vi "Process.vi"() -> ()   [LabVIEW 2020, in "RTAF.lvlib" / "System Status Actor.lvclass"]
uses:
  System Status Actor.lvclass
  Status.ctl
  Total Used Free MB.ctl
  Base Actor/Actor/Actor.lvclass/Actor.ctl
  Base Actor/Sequencer/Sequencer.lvclass/Sequencer.ctl
  System Status Actor.lvclass/System Status Actor.ctl
  C:/dev/PGS/2001 - TBCM/Source/RT/RTAF/Source/RTAF/Actors/Base Actor/Actor/Actor.lvclass
  API/System Status Actor API.lvclass
  <vilib>/Utility/High Resolution Relative Seconds.vi
  Global References.vi
  Base Actor/Actor/Actor.lvclass
  C:/dev/PGS/2001 - TBCM/Source/RT/RTAF/Source/RTAF/Actors/System Status/Actor/System Status Actor.lvclass
  RTAF.lvlib
panel:
  out "Status":T1 {"Uptime" format="%<%H:%M:%S%1u>t"}
  out "Iteration":i32
  in  "Tick Period [ms]":i32=5 min=2 step=1
  out "Tick Period [s]":dbl format="%.1p"
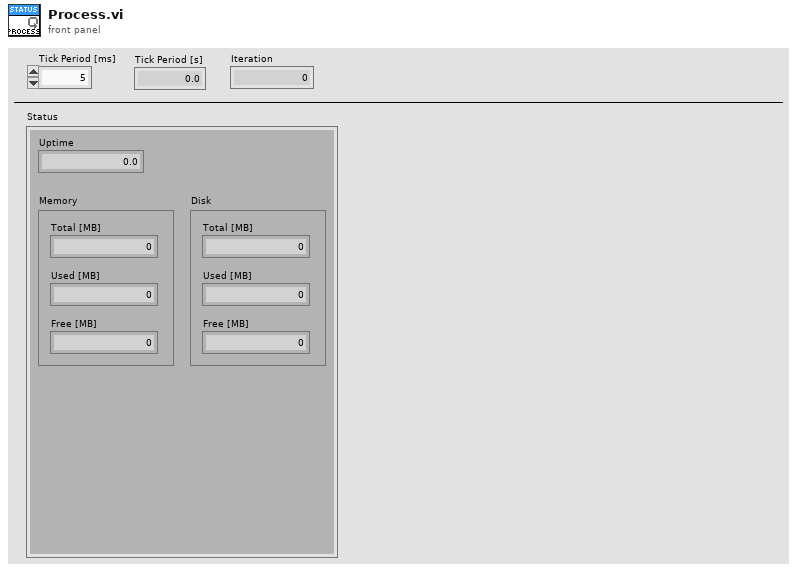
[diagram p1: front panel]
types:
  T1 = typedef "RTAF.lvlib/System Status Actor.lvclass/Status.ctl" = cluster{"Memory":T2, "Disk":T2, "Uptime":dbl}
  T2 = typedef "RTAF.lvlib/System Status Actor.lvclass/Total Used Free MB.ctl" = cluster{"Total [MB]":dbl, "Used [MB]":dbl, "Free [MB]":dbl}
  T3 = typedef "RTAF.lvlib/System Status Actor.lvclass/Mailboxes.ctl" = cluster{"Instructions":refnum<event-registration>}
  T4 = enum32{"Invalid", "Standard", "Closed", "Hidden", "Minimized", "Maximized"}
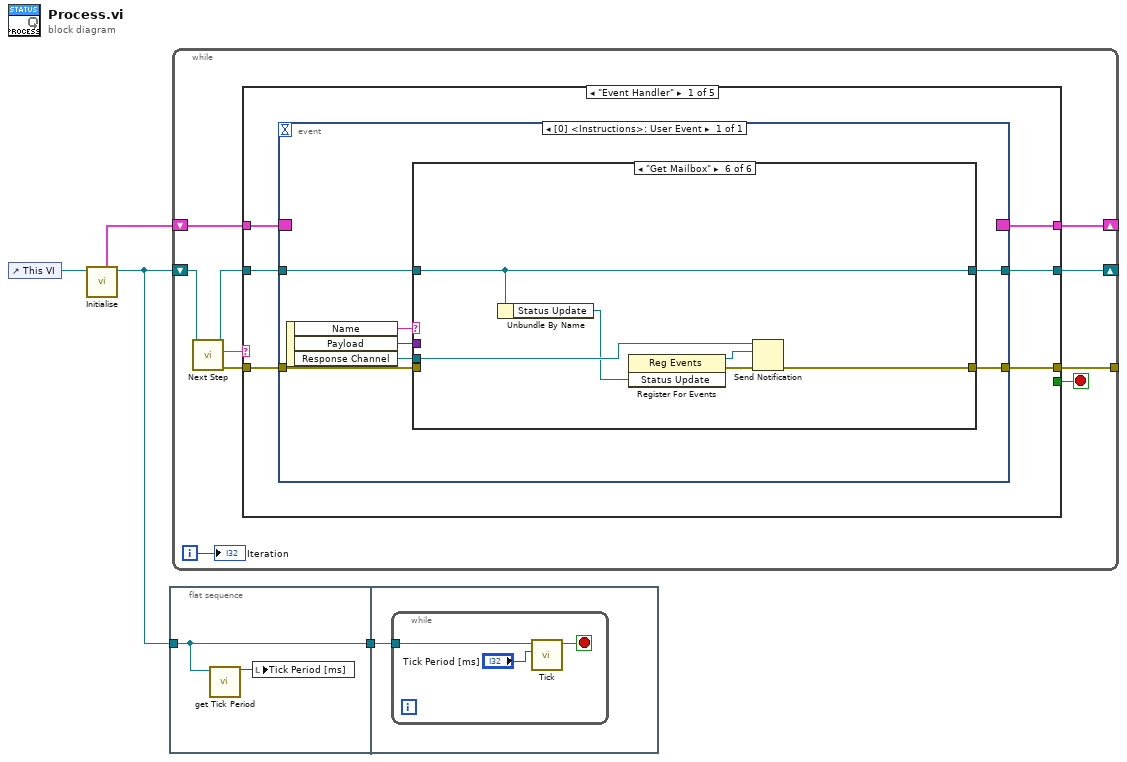
[diagram p0: block diagram]
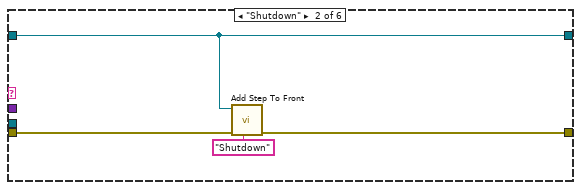
[diagram p3: hidden frame]
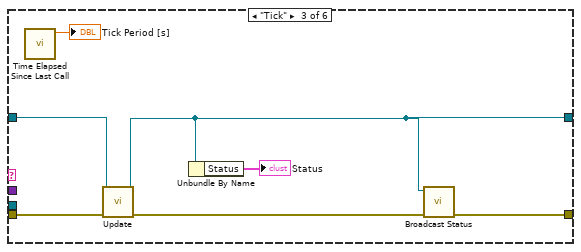
[diagram p4: hidden frame]
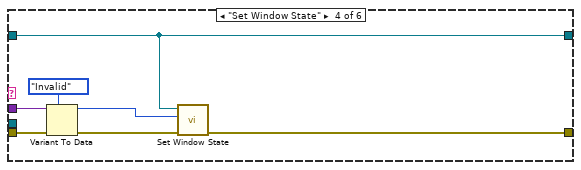
[diagram p5: hidden frame]
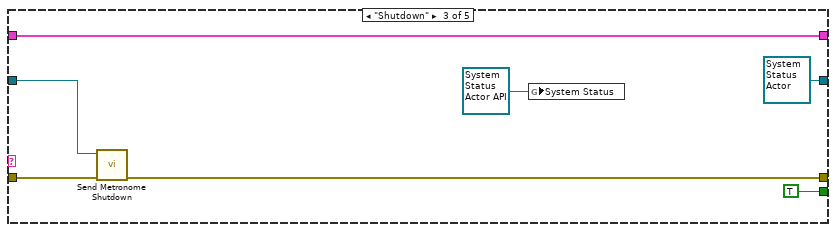
[diagram p8: hidden frame]
diagram:
  n1 = control-ref of="This VI"() -> (w3:refnum<vi>)
  n2 = call "Initialise.vi"("Process"=w3) -> ("Actor out"=w1:refnum<class "System Status Actor.lvclass">, "Mailboxes"=w2:T3)  [unwired: 8 in, 1 out]
  n3 = flat-sequence {
    tunnel: w1 -> [w6]
    tunnel: [w6] -> w4
    tunnel: w4 -> [w7]
    frame #0 {
      n4 = call "get Tick Period.vi"("Actor in"=w6) -> ("Tick Period [ms]"=w5:i32)  [unwired: 10 in]
      n5 = local write "Tick Period [ms]"(w5) -> ()
    }
    frame #1 {
      n6 = while {
        tunnel: w7 -> [w10]
        stop <- w8 stop-if-true
        n7 = call "Tick.vi"("Tick Period [ms]"="Tick Period [ms]", "Actor in"=w10) -> ("Shutdown"=w8:bool)  [unwired: 9 in]
      }
    }
  }
  n8 = while {
    shift-right: [w19] -> _
    shift-left: w1 -> [w16]
    tunnel: [w18] -> _
    shift-right: [w11] -> _
    shift-left: w2 -> [w20]
    i -> [w12]
    stop <- w13 stop-if-true
    n9 = call "Next Step.vi"("Actor in"=w16) -> ("error out"=w17:errorcluster, "Next Step"=w14:string, "Actor out"=w15:refnum<class "System Status Actor.lvclass">)  [unwired: 8 in]
    n10 = case shown="\"Event Handler\"" w14 {
      tunnel: w20 -> [w21 w61 w66 w71 w74]
      tunnel: [_ _ TRUE _ _] -> w13
      tunnel: w15 -> [w26 w63 w69 w73 w76]
      tunnel: [w25 w63 refnum<class "System Status Actor.lvclass"> refnum ("Actor out") w73 w76] -> w19
      tunnel: [w24 w62 w68 w72 w75] -> w18
      tunnel: w17 -> [w23 w62 w67 w72 w75]
      tunnel: [w22 w61 w66 w71 w74] -> w11
      frame "Event Handler" {
        n11 = event shown="[0] <Instructions>: User Event" {
          selector: w21 -> [_]
          dyn-events: [_] -> w22
          timeout: _ -> [_]
          tunnel: w26 -> [w31]
          tunnel: [w30] -> w25
          tunnel: [w28] -> w24
          tunnel: w23 -> [w27]
          event User Event {
            n12 = event-data() -> ("Name"=w33:string, "Payload"=w32:variant, "Response Channel"=w29:refnum<notifier>)  [unwired: 1 in]
            n13 = case shown="\"Get Mailbox\"" w33 {
              tunnel: w32 -> [_ _ _ w52 _ _]
              tunnel: w31 -> [w34 w38 w44 w48 w54 w60]
              tunnel: [w34 w38 w40 w48 w54 w60] -> w30
              tunnel: w29 -> [_ _ _ _ _ w59]
              tunnel: [_ w37 w41 w49 w53 w58] -> w28
              tunnel: w27 -> [_ w36 w43 w51 w53 _]
              frame Default {
              }
              frame "Shutdown" {
                n14 = call "Add Step To Front.vi"("Step Name"="Shutdown", "error in (no error)"=w36, "Actor in"=w38) -> ("error out"=w37:errorcluster)  [unwired: 8 in]
              }
              frame "Tick" {
                n15 = call "Time Elapsed Since Last Call.vi"() -> ("Time Elapsed Since Last Call [s]"=→"Tick Period [s]":dbl)  [unwired: 11 in]
                n16 = call "Update.vi"("error in (no error)"=w43, "System Status Actor in"=w44) -> ("error out"=w42:errorcluster, "System Status Actor out"=w40:refnum<class "System Status Actor.lvclass">)  [unwired: 8 in]
                n17 = Unbundle By Name(w40) -> ("Status"=→"Status":T1)
                n18 = call "Broadcast Status.vi"("error in (no error)"=w42, "Actor in"=w40) -> ("error out"=w41:errorcluster)  [unwired: 9 in]
              }
              frame "Set Window State" {
                n19 = Variant To Data(error in=w51, type=T4."Invalid", Variant=w52) -> (data=w47:T4, error out=w50:errorcluster)
                n20 = call "Set Window State.vi"("error in (no error)"=w50, "State"=w47, "Actor in"=w48) -> ("error out"=w49:errorcluster)  [unwired: 8 in]
              }
              frame "----------------------------------" {
              }
              frame "Get Mailbox" {
                n21 = Unbundle By Name(w60) -> ("Status Update"=w56:refnum<user-event>)
                n22 = register-events(w56) -> (reference out=w55:refnum<event-registration>, error out=w57:errorcluster)  [unwired: 2 in]
                n23 = Send Notification(notification=w55, notifier=w59, error in (no error)=w57) -> (error out=w58:errorcluster)  [unwired: 1 out]
              }
            }
          }
        }
      }
      frame "Error Handler" {
      }
      frame "Shutdown" {
        n24 = call "Send Metronome Shutdown.vi"("error in (no error)"=w67, "Actor in"=w69) -> ("error out"=w68:errorcluster)  [unwired: 9 in]
        n25 = global write "Global References.vi" "System Status"(refnum<class "System Status Actor API.lvclass"> refnum ("RTAF.lvlib:System Status Actor API.lvclass")) -> ()
      }
      frame "Unhandled Step", Default {
      }
      frame "-----------------------------------" {
      }
    }
    "Iteration" <- w12
  }
